vi "To Variant.vi"(8 "error in (no error)":errorcluster, 11 "Abs_Extended Float in":refnum<class "Abs_Extended Float.lvclass">) -> (0 "error out":errorcluster, 2 "Variant":variant, 3 "Abs_Extended Float out":refnum<class "Abs_Extended Float.lvclass">)   [LabVIEW 2021, in "Abs_Extended Float.lvclass"]
uses:
  Abs_Extended Float.lvclass
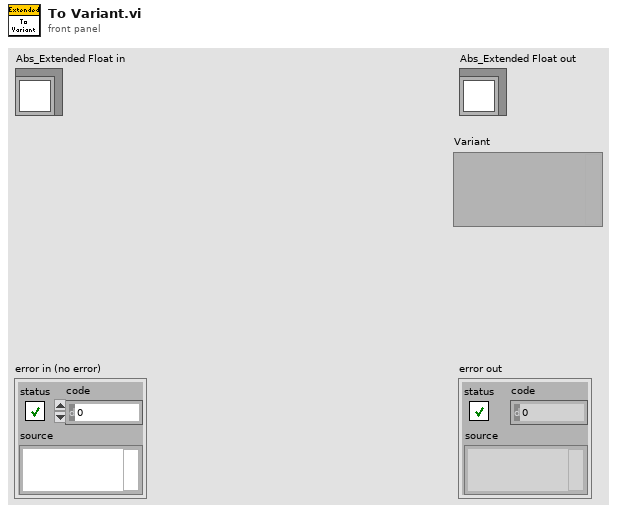
[diagram p1: front panel]
types:
  T1 = typedef "Abs_Extended Float.lvclass/Type.ctl" = ext
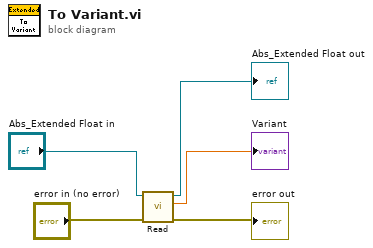
[diagram p0: block diagram]
diagram:
  n1 = call-dynamic "Read.vi"("error in (no error)"="error in (no error)", "Double Float.lvclass_340760 in"="Abs_Extended Float in") -> ("error out"=→"error out":errorcluster, "Value"=→"Variant":T1, "Double Float.lvclass_340760 out"=→"Abs_Extended Float out":refnum<class "Abs_Extended Float.lvclass">)  [unwired: 7 in]
